vi "Resolution Check.vi"(8 "error in":errorcluster, 9 "new list in":T1[](array[typedef]) {"Creation Date" format="%<%x>T"; "Last Updated" format="%<%x>T"}, 10 "VI in":refnum<vi>, 11 "SR List in":T1[](array[typedef]) {"Creation Date" format="%<%x>T"; "Last Updated" format="%<%x>T"}) -> (0 "error out":errorcluster, 1 "new list out":T1[](array[typedef]) {"Creation Date" format="%<%x>T"; "Last Updated" format="%<%x>T"}, 3 "list out":T1[](array[typedef]) {"Creation Date" format="%<%x>T"; "Last Updated" format="%<%x>T"})   [LabVIEW 2018]
uses:
  SR Cluster.ctl
  SR Status.ctl
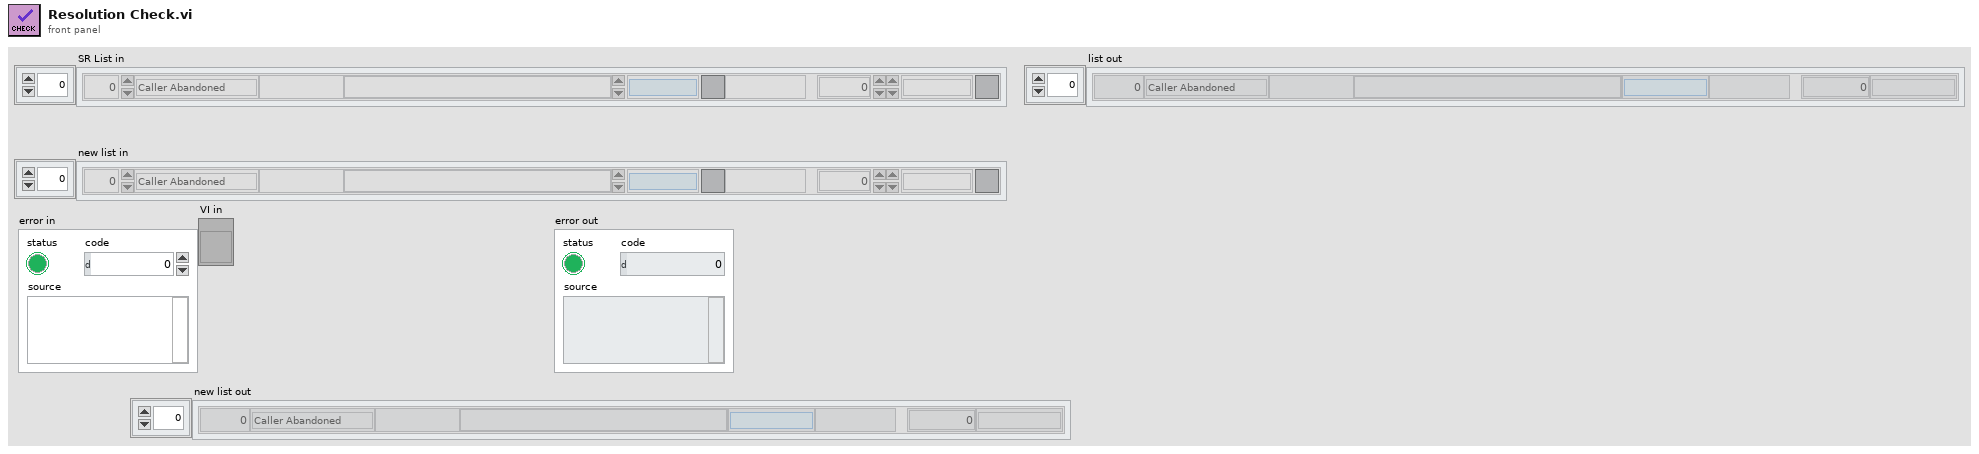
[diagram p1: front panel]
types:
  T1 = typedef "SR Cluster.ctl" = cluster{"SR Number":i32, "SR Status":T2, "SR Type":string, "Summary":string, "Last Updated":timestamp, "Service Level":string, "Days Open":dbl, "Creation Date":timestamp}
  T2 = typedef "SR Status.ctl" = enum16{"Caller Abandoned", "Created in Error", "Expired", "Forum Resolved AE", "Forum Resolved Customer", "IN WORK", "IN WORK Collab with AES", "IN WORK Collab with PSE", "IN WORK Collab with SE", "IN WORK Customer Added Note", "IN WORK Escalation", "IN WORK Wait on Customer", "Open", "Potentially Resolved", "Presumed Resolved", "RMA Approved for Return", "Resolved", "Passed Off"}
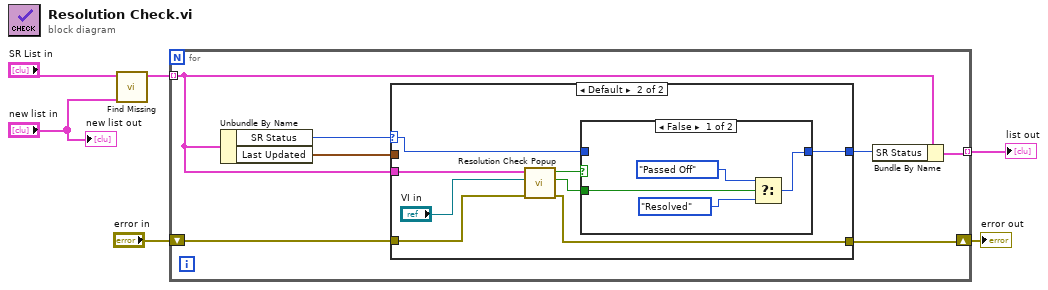
[diagram p0: block diagram]
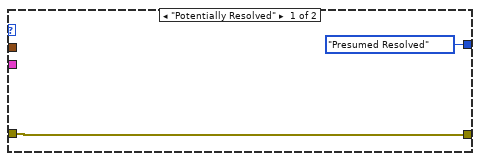
[diagram p2: hidden frame]
diagram:
  n1 = call "Find Missing.vi"("new list in"="new list in", "SR List in"="SR List in") -> ("missing list out"=w4:T1[])  [unwired: 9 in]
  n2 = for {
    tunnel: w4 -> [w7] mode=indexing
    tunnel: [w13] -> w3 mode=indexing
    shift-right: [w9] -> w1
    shift-left: "error in" -> [w10]
    n3 = Unbundle By Name(w7) -> ("SR Status"=w12:T2, "Last Updated"=w11:timestamp)
    n4 = case shown="Default" w12 {
      selector: w12 -> [_ w21]
      tunnel: w11 -> [_ _]
      tunnel: w10 -> [w15 w20]
      tunnel: [w15 w19] -> w9
      tunnel: [SR_Status."Presumed Resolved" ("SR Status") w18] -> w8
      tunnel: w7 -> [_ w17]
      frame "Potentially Resolved" {
      }
      frame Default {
        n5 = call "Resolution Check Popup.vi"("error in"=w20, "VI in"="VI in", "SR for Check"=w17) -> ("error out"=w19:errorcluster, "Passed Off?"=w23:bool, "Window Closed?"=w22:bool)  [unwired: 6 in]
        n6 = case shown="False" w22 {
          tunnel: [w27 w28] -> w18
          tunnel: w23 -> [w26 _]
          tunnel: w21 -> [_ w28]
          frame False {
            n7 = Select(t=SR_Status."Passed Off" ("SR Status"), s=w26, f=SR_Status."Resolved" ("SR Status")) -> (s? t:f=w27:T2)
          }
          frame True {
          }
        }
      }
    }
    n8 = Bundle By Name(cluster=w7, "SR Status"=w8) -> (w13:T1)
  }
  "list out" <- w3
  "error out" <- w1
  "new list out" <- "new list in"
